vi "Destroy.vi"(8 "error in (no error)":errorcluster, 11 "XRay CArm in":refnum<class "XRay CArm.lvclass">) -> (0 "error out":errorcluster, 3 "XRay CArm out":refnum<class "XRay CArm.lvclass">)   [LabVIEW 2026, in "XRay CArm.lvclass"]
uses:
  XRay CArm.lvclass
  XRay CArm.lvclass/XRay CArm.ctl
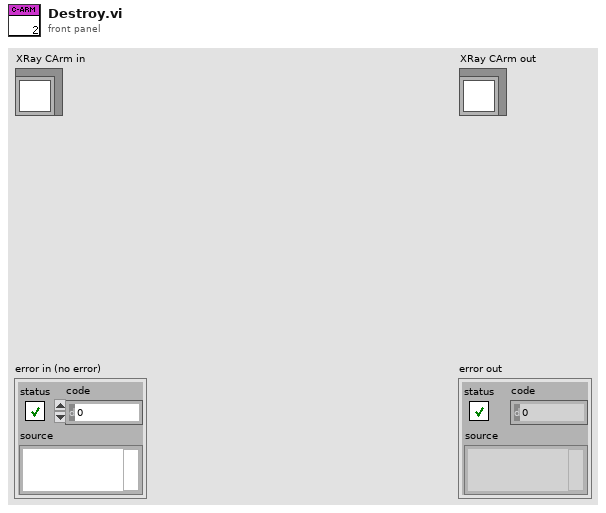
[diagram p1: front panel]
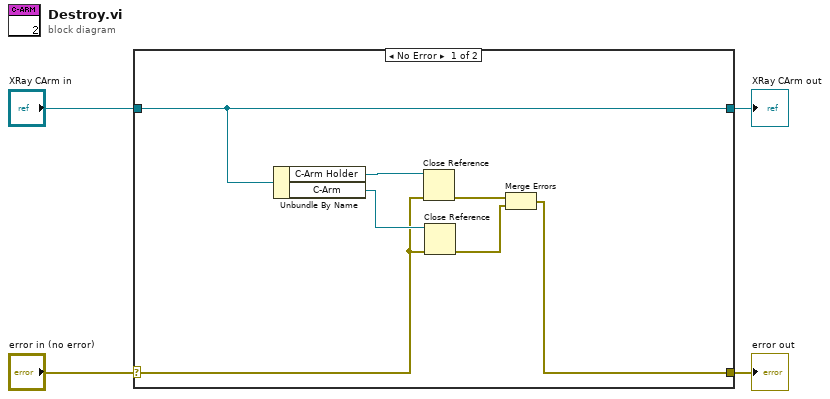
[diagram p0: block diagram]
diagram:
  n1 = case shown="No Error" "error in (no error)" {
    selector: "error in (no error)" -> [w8 w13]
    tunnel: [w5 w13] -> w3
    tunnel: [w11 w12] -> w1
    tunnel: "XRay CArm in" -> [w11 w12]
    frame No Error {
      n2 = Unbundle By Name(w11) -> ("C-Arm Holder"=w10:refnum<vi>, "C-Arm"=w9:refnum<vi>)
      n3 = Close Reference(reference=w10, error in (no error)=w8) -> (error out=w7:errorcluster)
      n4 = Close Reference(reference=w9, error in (no error)=w8) -> (error out=w6:errorcluster)
      n5 = Merge Errors(w7, w6) -> (w5:errorcluster)
    }
    frame Error {
    }
  }
  "error out" <- w3
  "XRay CArm out" <- w1
